vi "merFISH_hybridization_pump.vi"(2 "error in":errorcluster, 3 "input data cluster":T1, 4 "queue pump":refnum<queue>) -> (0 "error out":errorcluster)   [LabVIEW 2015]
uses:
  CONTROLS/Q_PUMP_element.ctl
  GLOBAL/Global_ABORT.vi
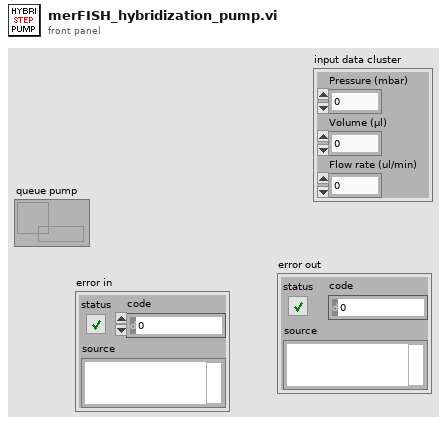
[diagram p1: front panel]
types:
  T1 = cluster{"Pressure (mbar)":i32, "Volume (µl)":i32, "Flow rate (ul/min) ":i32}
  T2 = typedef "Q_PUMP_element.ctl" = cluster{"variant":variant, "Instruction":enum16{"PUMP_idle", "PUMP_initialize", "PUMP_error", "PUMP_security_stop", "PUMP_read_pressure", "PUMP_change_pressure", "PUMP_init_merFISH", "PUMP_change_presure_merFISH", "PUMP_zero_pressure_merFISH", "PUMP_close_merFISH", "PUMP_stop"}}
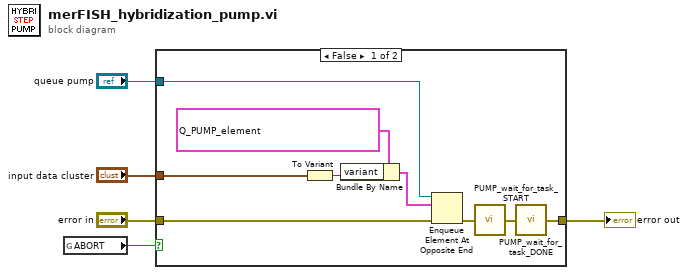
[diagram p0: block diagram]
diagram:
  n1 = global read "Global_ABORT.vi" "ABORT"() -> (w3:bool)
  n2 = case shown="False" w3 {
    tunnel: [w14 w15] -> w5
    tunnel: "queue pump" -> [w13 _]
    tunnel: "input data cluster" -> [w7 _]
    tunnel: "error in" -> [w6 w15]
    frame False {
      n3 = To Variant(anything=w7) -> (Variant=w12:variant)
      n4 = Bundle By Name(cluster=T2 {"variant"=variant, "Instruction"=enum."PUMP_change_presure_merFISH"} ("element"), "variant"=w12) -> (w10:T2)
      n5 = Enqueue Element At Opposite End(queue=w13, element=w10, error in (no error)=w6) -> (error out=w9:errorcluster)  [unwired: 1 in, 2 out]
      n6 = call "PUMP_wait_for_task_START.vi"("error in"=w9) -> ("error out"=w8:errorcluster)
      n7 = call "PUMP_wait_for_task_DONE.vi"("error in"=w8) -> ("error out"=w14:errorcluster)
    }
    frame True {
    }
  }
  "error out" <- w5
